vi "Connect.vi"(8 "error in (no error)":errorcluster, 11 "Arduino in":refnum<class "Arduino.lvclass">) -> (0 "error out":errorcluster, 3 "Arduino out":refnum<class "Arduino.lvclass">)   [LabVIEW 2016, in "Arduino.lvclass"]
uses:
  Arduino.lvclass
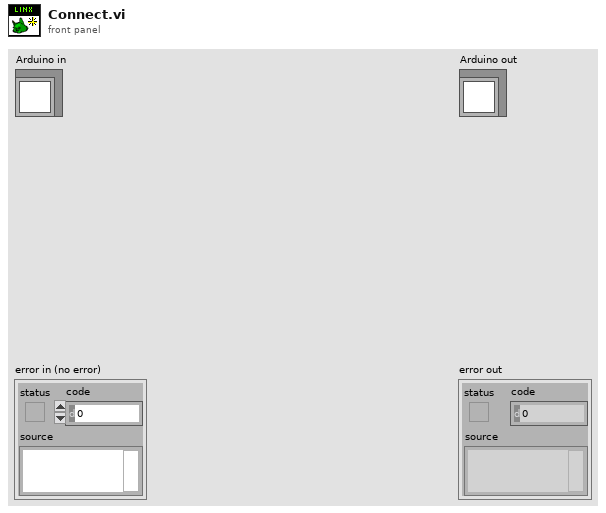
[diagram p1: front panel]
types:
  T1 = typedef "LMH-LINX.lvlib/LINX Ref.ctl" = cluster{"IO":T2, "Interface":T3, "LINX Device Config":T4}
  T2 = typedef "LMH-LINX.lvlib/Platform.ctl" = enum16{"Remote", "Local"}
  T3 = typedef "LMH-LINX.lvlib/Interface.ctl" = enum16{"Serial", "TCP"}
  T4 = typedef "LMH-LINX.lvlib/Device.lvlib/LINX Device Config.ctl" = cluster{"Interface":T3, "COM Port":refnum<visa-resource-name>, "TCP Configuration":T5, "Device Family":u8, "Device ID":u8, "Device Name":string, "TCP Ref":refnum<k5>, "Channels":T6}
  T5 = typedef "LMH-LINX.lvlib/Device.lvlib/TCP Config.ctl" = cluster{"IP Address":string, "Port":u16}
  T6 = typedef "LMH-LINX.lvlib/Channels.ctl" = cluster{"DI":u8[], "DO":u8[], "AI":u8[], "AO":u8[], "PWM":u8[], "QE":u8[], "UART":u8[], "I2C 2":u8[], "SPI":u8[], "CAN":u8[], "Servo":u8[], "AI Ref (V)":dbl, "AI Resolution (Bits)":u8, "AO Ref (V)":dbl, "AO Resolution (Bits)":u8}
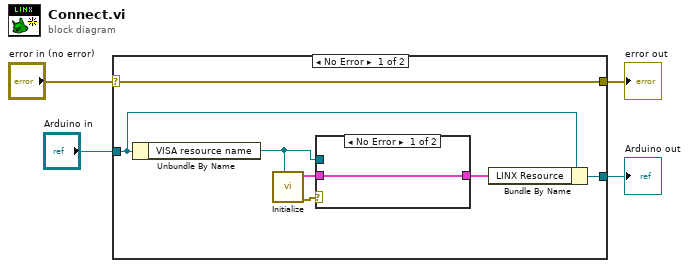
[diagram p0: block diagram]
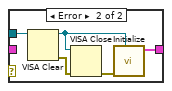
[diagram p2: hidden frame]
diagram:
  n1 = case shown="No Error" "error in (no error)" {
    selector: "error in (no error)" -> [w11 w19]
    tunnel: [w11 w19] -> w3
    tunnel: [w7 w18] -> w1
    tunnel: "Arduino in" -> [w6 w18]
    frame No Error {
      n2 = Unbundle By Name(w6) -> ("VISA resource name"=w5:refnum<visa-resource-name>)
      n3 = call <vilib>:"Initialize.vi"("Serial Port"=w5) -> ("Error Out"=w9:errorcluster, "LINX Resource"=w10:T1)  [unwired: 8 in, 1 out]
      n4 = case shown="No Error" w9 {
        tunnel: w10 -> [w12 _]
        tunnel: [w12 w16] -> w8
        tunnel: w5 -> [_ w13]
        frame No Error {
        }
        frame Error {
          n5 = VISA Clear(VISA resource name=w13) -> (VISA resource name out=w15:refnum<visa-resource-name>, error out=w14:errorcluster)  [unwired: 1 in]
          n6 = VISA Close(VISA resource name=w15, error in (no error)=w14) -> (error out=w17:errorcluster)
          n7 = call <vilib>:"Initialize.vi"("Serial Port"=w15, "Error In"=w17) -> ("LINX Resource"=w16:T1)  [unwired: 7 in, 2 out]
        }
      }
      n8 = Bundle By Name(cluster=w6, "LINX Resource"=w8) -> (w7:refnum<class "Arduino.lvclass">)
    }
    frame Error {
    }
  }
  "error out" <- w3
  "Arduino out" <- w1
